vi "gRPC Client Test.vi"() -> ()   [LabVIEW 2021, in "streamtest_client.lvlib"]
uses:
  streamtest_client.lvlib
  <vilib>/gRPC/LabVIEW gRPC Library/grpc-lvsupport-release.lvlib
  <vilib>/gRPC/LabVIEW gRPC Library/Shared/Any.ctl
  RPC Messages/streamtest_StreamData.ctl
panel:
  in  "milliseconds to wait":u32=50
  out "error out 3":errorcluster
  in  "Boolean":bool
  out "error out 2":errorcluster
  out "Success":bool
  out "Response Data":T1
  out "errorDetails":T2
  out "error out":errorcluster
  in  "address":string="localhost:50051"
  in  "stop":bool
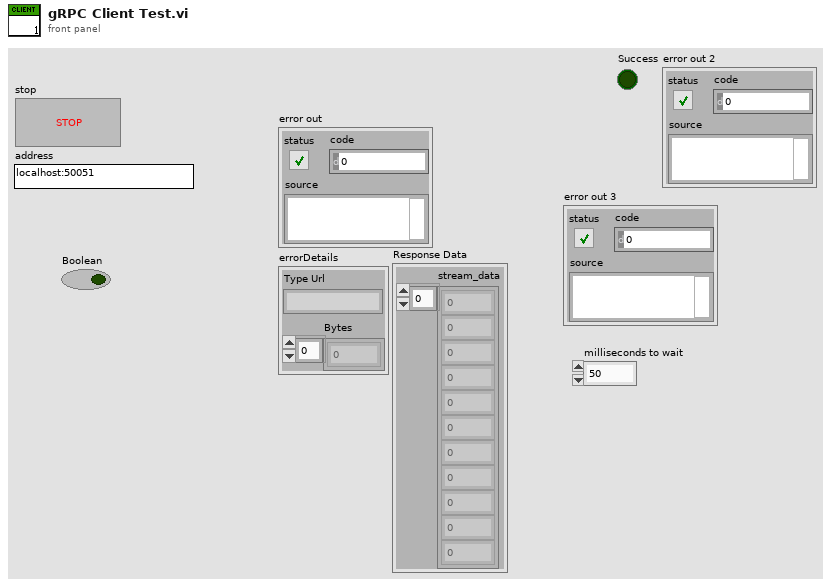
[diagram p1: front panel]
types:
  T1 = typedef "streamtest_client.lvlib/streamtest_StreamData.ctl" = cluster{"stream_data":u8[]}
  T2 = typedef "grpc-lvsupport-release.lvlib/Any.ctl" = cluster{"Type Url":string, "Bytes":u8[]}
  T3 = typedef "grpc-lvsupport-release.lvlib/grpcId.ctl" = u64
  T4 = typedef "Call ID.ctl" = cluster{"Call Id":T3, "occurrence":refnum<k4>}
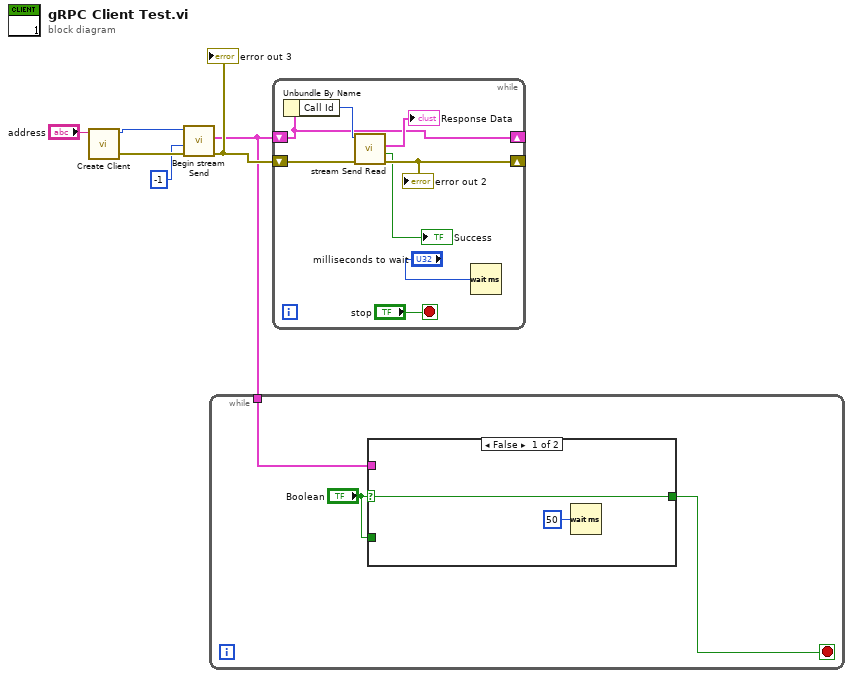
[diagram p0: block diagram]
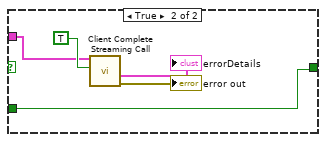
[diagram p2: hidden frame]
diagram:
  n1 = call "Create Client.vi"("address"="address") -> ("error out"=w5:errorcluster, "gRPC ID Out"=w6:T3)  [unwired: 9 in]
  n2 = call "Begin stream Send.vi"("error in"=w5, "timeout (ms)"=-1, "gRPC ID"=w6) -> ("error out"=w4:errorcluster, "Optimized Streaming"=w1:T4)  [unwired: 6 in, 1 out]
  "error out 3" <- w4
  n3 = while {
    tunnel: w1 -> [w7]
    stop <- w9 stop-if-true
    n4 = case shown="False" "Boolean" {
      selector: "Boolean" -> [w10 _]
      tunnel: [w10 w13] -> w9
      tunnel: "Boolean" -> [_ w13]
      tunnel: w7 -> [_ w12]
      frame False {
        n5 = Wait (ms)(milliseconds to wait=u32 50) -> ()  [unwired: 1 out]
      }
      frame True {
        n6 = call <vilib>:"Client Complete Streaming Call.vi"("Cancel All Reads (T)"=TRUE ("Cancel All Reads (F)"), "Optimized Streaming in"=w12) -> ("error out"=→"error out":errorcluster, "errorDetails"=→"errorDetails":T2)  [unwired: 8 in]
      }
    }
  }
  n7 = while {
    shift-right: [w17] -> _
    shift-left: w1 -> [w17]
    shift-right: [w23] -> _
    shift-left: w4 -> [w24]
    stop <- "stop" stop-if-true
    n8 = Unbundle By Name(w17) -> ("Call Id"=w18:T3)
    n9 = call "stream Send Read.vi"("error in"=w24, "Call ID in"=w18) -> ("error out"=w23:errorcluster, "Success"=→"Success":bool, "Response Data"=→"Response Data":T1)  [unwired: 6 in, 1 out]
    "error out 2" <- w23
    n10 = Wait (ms)(milliseconds to wait="milliseconds to wait") -> ()  [unwired: 1 out]
  }
